vi "MoveBySteps.vi"(6 "Direction":enum16{"Forward", "Backwards"}(ring), 7 "Polarity":enum16{"Positive", "Negative"}(ring), 8 "error in (no error)":errorcluster, 9 "Speed":u32, 10 "Steps":u32) -> (0 "error out":errorcluster)   [LabVIEW 2023, in "TranslationStages.lvclass"]
uses:
  TranslationStages.lvclass
panel:
  in  "TranslationStages.lvclass":refnum<class "TranslationStages.lvclass">
  out "TranslationStages.lvclass":refnum<class "TranslationStages.lvclass">
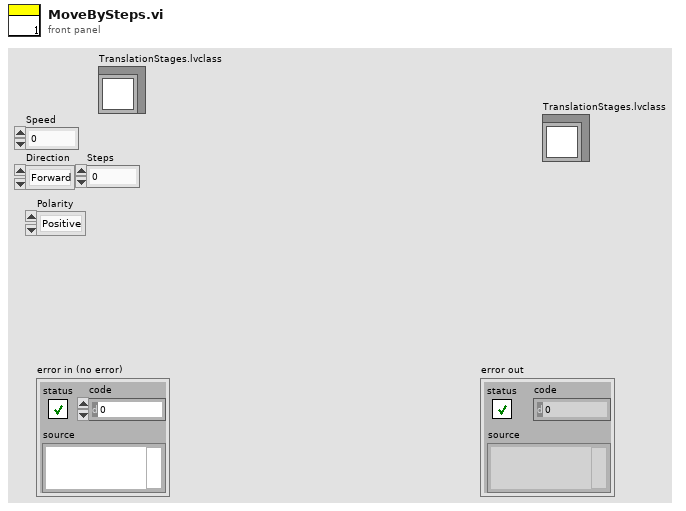
[diagram p1: front panel]
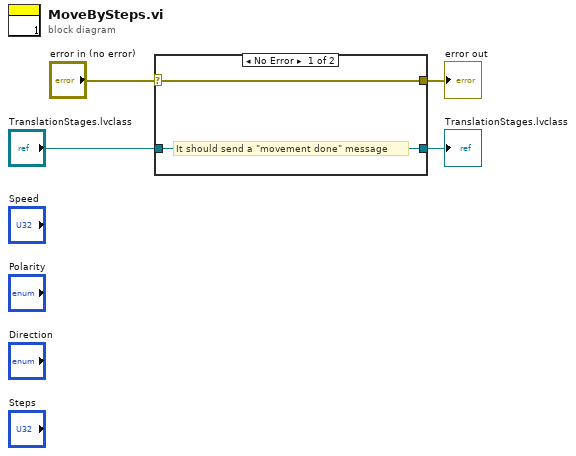
[diagram p0: block diagram]
diagram:
  n1 = case shown="No Error" "error in (no error)" {
    selector: "error in (no error)" -> [w5 w8]
    tunnel: [w5 w8] -> w3
    tunnel: [w6 w7] -> w2
    tunnel: "TranslationStages.lvclass" -> [w6 w7]
    frame No Error {
      # "It should send a \"movement done\" message"
    }
    frame Error {
    }
  }
  "error out" <- w3
  "TranslationStages.lvclass" <- w2
